vi "Affichage - 2 cam - 2P - 2.vi"(6 "Couleur rectangle 2":u32(colorbox)=16775680, 7 "Image 2D 2":picture, 8 "Couleur rectangle":u32(colorbox)=16775680, 9 "Caméra D":T1, 10 "Choix cam":u16, 11 "Caméra G":T1) -> (2 "Image 2D":picture)   [LabVIEW 2013]
panel:
  # "Affichage"
  # "Pour un rectangle"
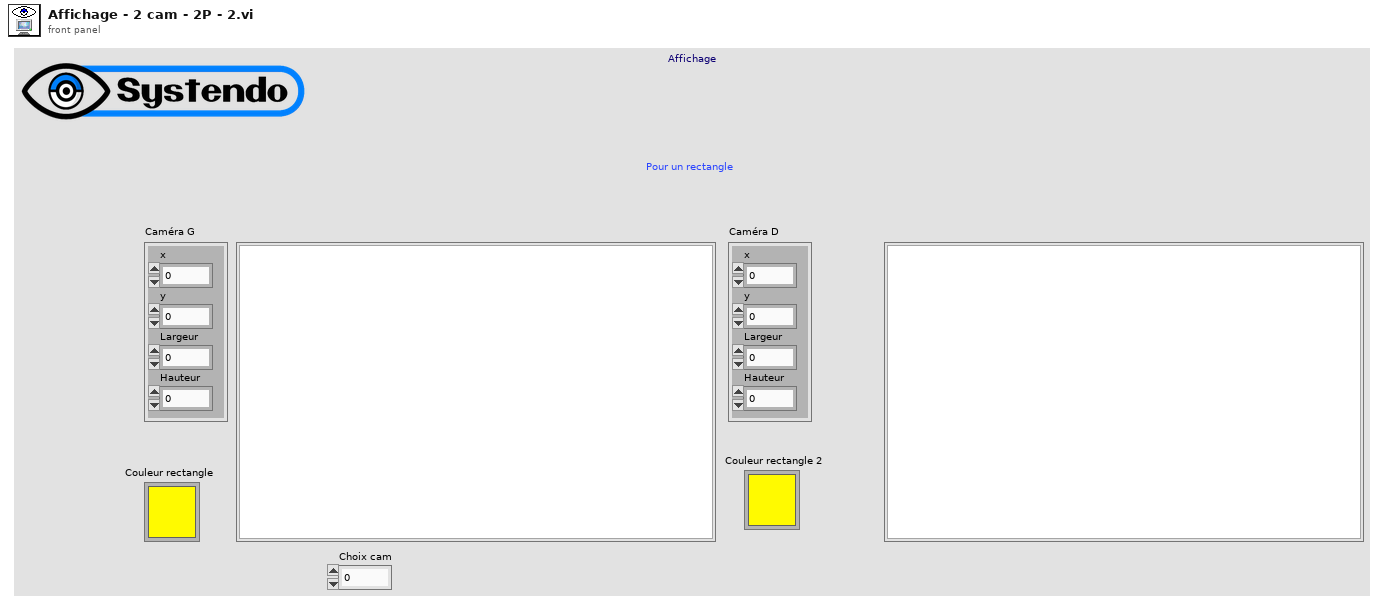
[diagram p1: front panel]
types:
  T1 = cluster{"x":i16, "y":i16, "Largeur":i16, "Hauteur":i16}
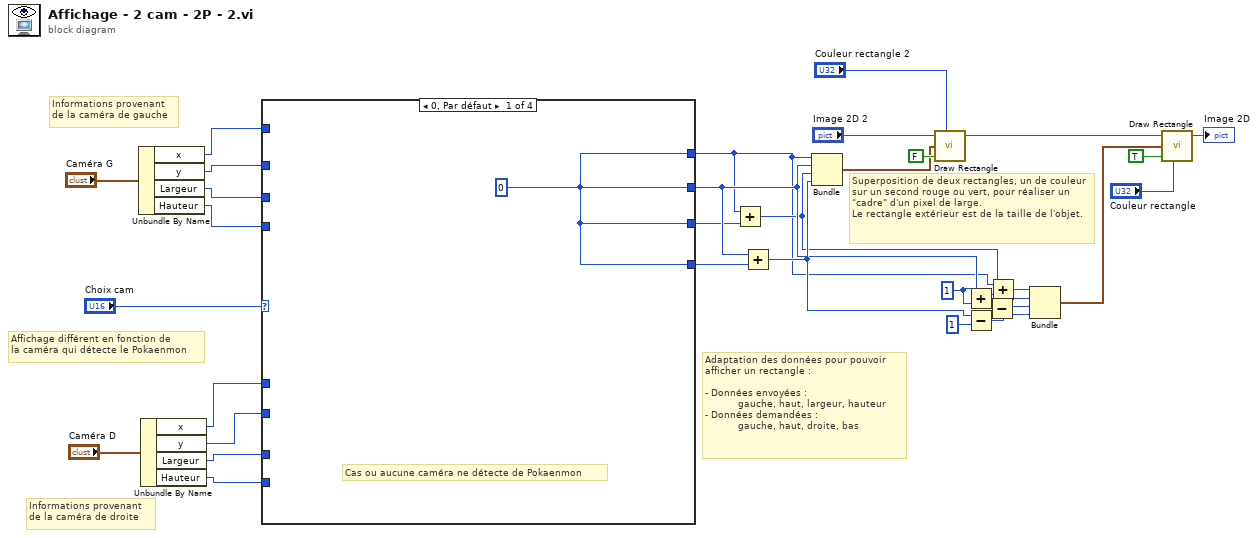
[diagram p0: block diagram]
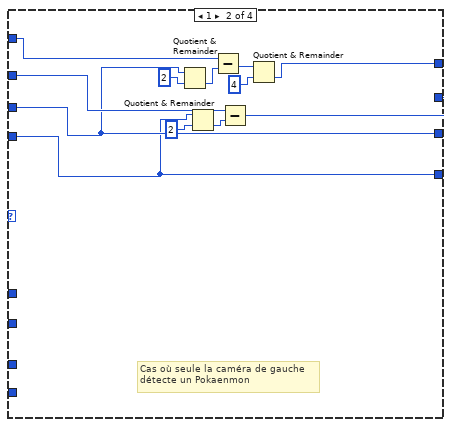
[diagram p2: hidden frame]
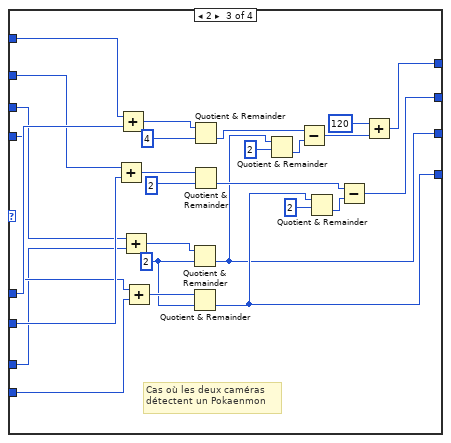
[diagram p3: hidden frame]
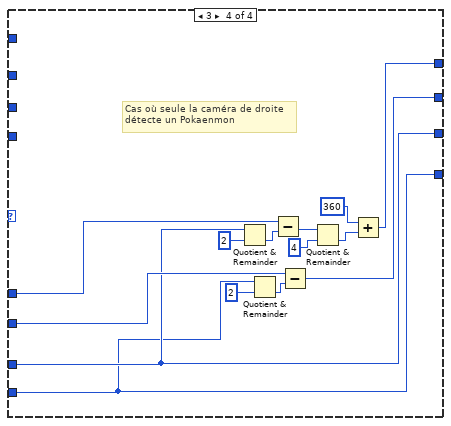
[diagram p4: hidden frame]
diagram:
  w11 = i16 1 ("y")
  w8 = i16 1 ("y")
  # "Superposition de deux rectangles, un de couleur sur un second rouge ou vert, pour réaliser un \"cadre\" d'un pixel de large.\nLe rectangle extérieur est de la taille de l'objet."
  # "Adaptation des données pour pouvoir\nafficher un rectangle :\n\n- Données envoyées :\n           gauche, haut, largeur, hauteur\n- Données demandées :\n           gauche, haut, droite, bas"
  # "Informations provenant\nde la caméra de droite"
  # "Informations provenant\nde la caméra de gauche"
  # "Affichage différent en fonction de\nla caméra qui détecte le Pokaenmon"
  n1 = Unbundle By Name("Caméra G") -> ("x"=w24:i16, "y"=w23:i16, "Largeur"=w22:i16, "Hauteur"=w21:i16)
  n2 = Unbundle By Name("Caméra D") -> ("x"=w17:i16, "y"=w18:i16, "Largeur"=w19:i16, "Hauteur"=w20:i16)
  n3 = case shown="0, Par défaut" "Choix cam" {
    tunnel: [w33 w37 w55 w82] -> w28
    tunnel: [w33 w43 w54 w84] -> w31
    tunnel: [w33 w41 w46 w77] -> w27
    tunnel: [w33 w35 w52 w74] -> w30
    tunnel: w17 -> [_ _ w65 w85]
    tunnel: w18 -> [_ _ w63 w86]
    tunnel: w19 -> [_ _ w60 w77]
    tunnel: w20 -> [_ _ w62 w74]
    tunnel: w21 -> [_ w35 w61 _]
    tunnel: w22 -> [_ w41 w59 _]
    tunnel: w23 -> [_ w44 w64 _]
    tunnel: w24 -> [_ w45 w66 _]
    frame 0, Default {
      w33 = 0
      # "Cas ou aucune caméra ne détecte de Pokaenmon"
    }
    frame 1 {
      # "Cas où seule la caméra de gauche\ndétecte un Pokaenmon"
      n4 = Quotient & Remainder(x=w41, y=u16 2) -> (floor(x/y)=w40:u16)  [unwired: 1 out]
      n5 = Quotient & Remainder(x=w35, y=u16 2) -> (floor(x/y)=w34:u16)  [unwired: 1 out]
      n6 = Subtract(x=w45, y=w40) -> (x-y=w38:u16)
      n7 = Subtract(x=w44, y=w34) -> (x-y=w43:u16)
      n8 = Quotient & Remainder(x=w38, y=u16 4) -> (floor(x/y)=w37:u16)  [unwired: 1 out]
    }
    frame 2 {
      w67 = i16 2 ("y")
      # "Cas où les deux caméras\ndétectent un Pokaenmon"
      n9 = Add(x=w64, y=w63) -> (x+y=w71:i16)
      n10 = Add(x=w66, y=w65) -> (x+y=w72:i16)
      n11 = Add(x=w59, y=w60) -> (x+y=w69:i16)
      n12 = Add(x=w61, y=w62) -> (x+y=w68:i16)
      n13 = Quotient & Remainder(x=w69, y=w67) -> (floor(x/y)=w46:i16)  [unwired: 1 out]
      n14 = Quotient & Remainder(x=w68, y=w67) -> (floor(x/y)=w52:i16)  [unwired: 1 out]
      n15 = Quotient & Remainder(x=w72, y=i16 4) -> (floor(x/y)=w48:i16)  [unwired: 1 out]
      n16 = Quotient & Remainder(x=w71, y=i16 2) -> (floor(x/y)=w57:i16)  [unwired: 1 out]
      n17 = Quotient & Remainder(x=w46, y=u16 2) -> (floor(x/y)=w49:u16)  [unwired: 1 out]
      n18 = Subtract(x=w48, y=w49) -> (x-y=w47:u16)
      n19 = Quotient & Remainder(x=w52, y=u16 2) -> (floor(x/y)=w51:u16)  [unwired: 1 out]
      n20 = Subtract(x=w57, y=w51) -> (x-y=w54:u16)
      n21 = Add(x=u16 120, y=w47) -> (x+y=w55:u16)
    }
    frame 3 {
      # "Cas où seule la caméra de droite\ndétecte un Pokaenmon"
      n22 = Quotient & Remainder(x=w77, y=u16 2) -> (floor(x/y)=w76:u16)  [unwired: 1 out]
      n23 = Quotient & Remainder(x=w74, y=u16 2) -> (floor(x/y)=w73:u16)  [unwired: 1 out]
      n24 = Subtract(x=w85, y=w76) -> (x-y=w80:u16)
      n25 = Subtract(x=w86, y=w73) -> (x-y=w84:u16)
      n26 = Quotient & Remainder(x=w80, y=u16 4) -> (floor(x/y)=w79:u16)  [unwired: 1 out]
      n27 = Add(x=u16 360, y=w79) -> (x+y=w82:u16)
    }
  }
  n28 = Add(x=w28, y=w27) -> (x+y=w29:i32)
  n29 = Add(x=w31, y=w30) -> (x+y=w32:i32)
  n30 = Bundle(w28, w31, w29, w32) -> (w3:cluster{i32, i32, i32, i32})  [unwired: 1 in]
  n31 = call <vilib>:"Draw Rectangle.vi"("picture"="Image 2D 2", "rect"=w3, "fill?(F)"=FALSE, "color(black)"="Couleur rectangle 2") -> ("new picture"=w14:picture)  [unwired: 5 in]
  n32 = Add(x=w31, y=w8) -> (x+y=w7:i32)
  n33 = Subtract(x=w32, y=w11) -> (x-y=w10:i32)
  n34 = Subtract(x=w29, y=w11) -> (x-y=w9:i32)
  n35 = Add(x=w28, y=w8) -> (x+y=w6:i32)
  n36 = Bundle(w6, w7, w9, w10) -> (w12:cluster{i32, i32, i32, i32})  [unwired: 1 in]
  n37 = call <vilib>:"Draw Rectangle.vi"("picture"=w14, "rect"=w12, "fill?(F)"=TRUE, "color(black)"="Couleur rectangle") -> ("new picture"=→"Image 2D":picture)  [unwired: 5 in]
